vi "Dallas digital out toggle.vi"() -> ()   [LabVIEW 2009]
uses:
  <vilib>/DAQmx/write.llb/DAQmx Write (Digital Bool 1Line 1Point).vi
  <vilib>/DAQmx/create/channels.llb/DAQmx Create Channel (DO-Digital Output).vi
panel:
  in  "stop":bool
  in  "2":bool
  in  "1":bool
  in  "channel 0":bool
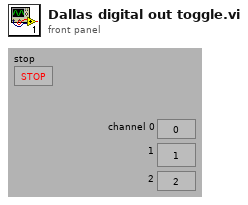
[diagram p1: front panel]
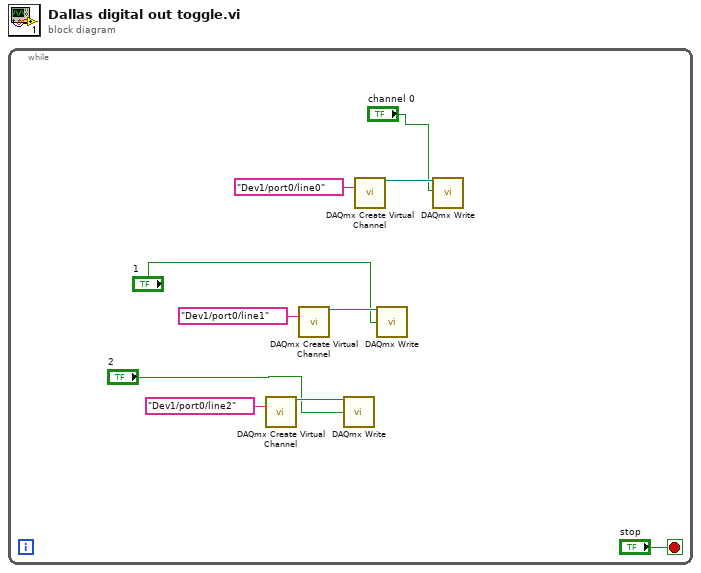
[diagram p0: block diagram]
diagram:
  n1 = while {
    stop <- "stop" stop-if-true
    n2 = call-poly <vilib>:"DAQmx Create Virtual Channel.vi"("lines"=tag "Dev1/port0/line2") -> ("task out"=w5:refnum<k21>)  [unwired: 5 in, 9 out]
    n3 = call-poly <vilib>:"DAQmx Create Virtual Channel.vi"("lines"=tag "Dev1/port0/line1") -> ("task out"=w7:refnum<k21>)  [unwired: 5 in, 9 out]
    n4 = call-poly <vilib>:"DAQmx Write.vi"("task/channels in"=w5, "data"="2") -> ()  [unwired: 2 in, 12 out]
    n5 = call-poly <vilib>:"DAQmx Create Virtual Channel.vi"("lines"=tag "Dev1/port0/line0") -> ("task out"=w9:refnum<k21>)  [unwired: 5 in, 9 out]
    n6 = call-poly <vilib>:"DAQmx Write.vi"("task/channels in"=w7, "data"="1") -> ()  [unwired: 2 in, 12 out]
    n7 = call-poly <vilib>:"DAQmx Write.vi"("task/channels in"=w9, "data"="channel 0") -> ()  [unwired: 2 in, 12 out]
  }
